vi "STEP SPEED SEQUENCE.vi"(8 "error in (no error)":errorcluster, 11 "main ref":T1) -> (0 "error out":errorcluster)   [LabVIEW 2025]
uses:
  controls/LAB-IQ UI Data.ctl
  Traction Loop/Traction Receipe Enum.ctl
  STEP SPEED SEQUENCE ENUM.ctl
  SWAY vi's/Sway Write enum.ctl
  LOAD CELL CODE/STEP LOAD SEQUENCE ENUM.ctl
  cef93557-1e48-4b46-994d-460df1ebe7ff.vi
  HEAVE vi's/Heave Write enum.ctl
panel:
  in  "Checkbox":bool
  out "ELAPSED TIMER":dbl
  out "Test Size":i32
  in  "Time Index":i32
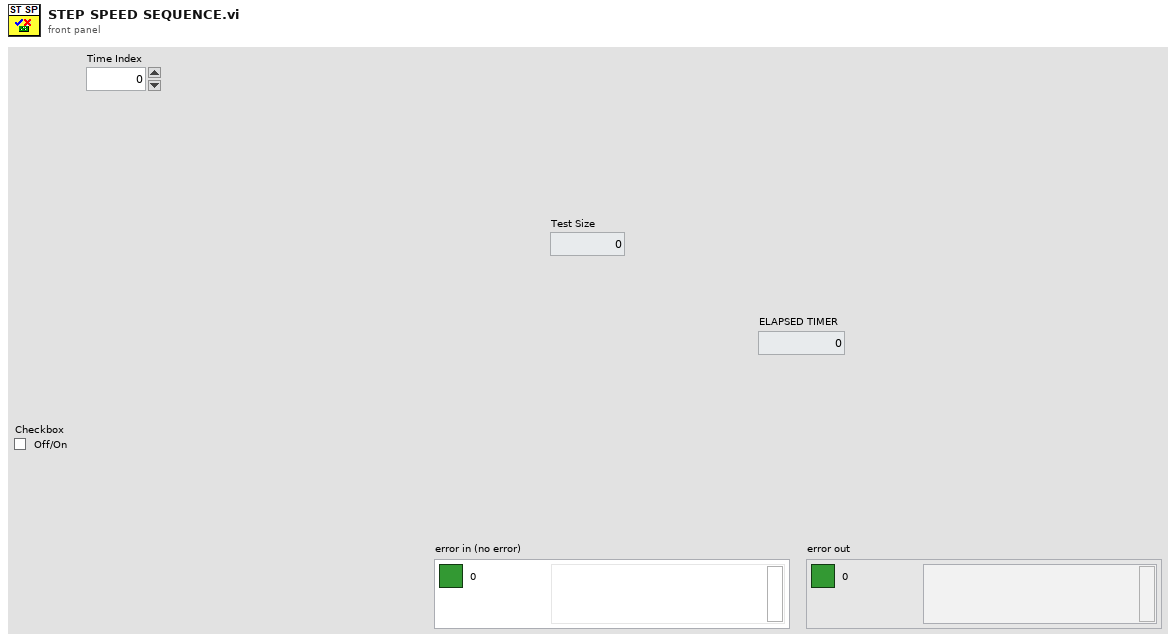
[diagram p1: front panel]
types:
  T1 = typedef "LAB-IQ UI Data.ctl" = cluster{"Main Home Screen":cluster{"GUI":refnum<vi>, "Platform Settings":refnum<vi>, "Configure":refnum<vi>, "Home":refnum<vi>, "EXIT":refnum<vi>, "service 2":refnum<vi>, "MainPage":refnum<vi>, "Analysis":refnum<vi>}, "Platform Settings":cluster{"mm/s  Surge":refnum<vi>, "Update Surge Speed":refnum<vi>, "Drive Error":refnum<vi>, "Disable Axis Jog Soft Limits":refnum<vi>, "mm/s  Sway":refnum<vi>, "Sway and Surge COM Status":refnum<vi>, "Heave COM Status":refnum<vi>, "Enable Platform":refnum<vi>, "Surge Forward Main":refnum<vi>, "Sway Right Main":refnum<vi>, "Sway Left Main":refnum<vi>, "Heave Down Main":refnum<vi>, "Heave Up main":refnum<vi>, "Update Sway Speed":refnum<vi>, "Update Heave Speed":refnum<vi>, "mm/s Heave":refnum<vi>, "mm/sec":refnum<vi>, "mm":refnum<vi>, "Surge Backward Main":refnum<vi>}, "Analysis Screen":cluster{"Analysis Home":refnum<vi>, "Surface Analysis":refnum<vi>, "Imaging":refnum<vi>, "Image Analysis":refnum<vi>, "Post Analysis":refnum<vi>}, "Config Screen":cluster{"Select Load Head":refnum<vi>, "Notes :":refnum<vi>, "FILE":refnum<vi>, "Sample ID :":refnum<vi>, "Operator ID :":refnum<vi>, "Operator Name :":refnum<vi>, "Auto":refnum<vi>}, "Motion Module":cluster{"zNL":refnum<vi>, "NL disp":refnum<vi>, "Rotary Tab":refnum<vi>, "Motion Direction:  3":refnum<vi>, "E.Velocity 2":refnum<vi>, "e.v/ssr 2":refnum<vi>, "Enter Fixed E.Velocity 2":refnum<vi>, "Enter Final SRR 2":refnum<vi>, "Enter initial SRR 2":refnum<vi>, "Enter Fixed SRR 2":refnum<vi>, "Enter the Final E.Velocity (m/s) 2":refnum<vi>, "Enter initial E.Velocity (m/s) 2":refnum<vi>, "Final Speed (RPM) 3":refnum<vi>, "Initial Speed (RPM) 2":refnum<vi>, "Enter the Final Velocity (m/s) 3":refnum<vi>, "Enter initial Velocity (m/s)  3":refnum<vi>, "Ramp Up 2":refnum<vi>, "TEST SELECTION":refnum<vi>, "SPEED SELECTION : ":refnum<vi>, "Angular Oscillation Set":refnum<vi>, "Traction":refnum<vi>, "Step Speed":refnum<vi>, "StepTable For Load-Speed":refnum<vi>, "StepTable For Speed":refnum<vi>, "Surge Forward MM":refnum<vi>, "Surge Backward MM":refnum<vi>, "M3 Image":refnum<vi>, "String 39":refnum<vi>, "Sway Left MM":refnum<vi>, "Sway Right MM":refnum<vi>, "Disable Axis Jog Soft Limits":refnum<vi>, "mm":refnum<vi>, "Heave Down MM":refnum<vi>, "Heave Up MM":refnum<vi>, "Wear Track Diameter (mm)":refnum<vi>, "Set WTD":refnum<vi>, "HomeScratch":refnum<vi>, "HomeRot":refnum<vi>, "PlaceModule":refnum<vi>, "Enter the Angle (Deg)":refnum<vi>, "Enter the Frequency (Hz)":refnum<vi>, "Motion Mode:":refnum<vi>, "LR Sway":refnum<vi>, "Rot Hor":refnum<vi>, "Scratch":refnum<vi>, "LR Cam":refnum<vi>, "MMBack":refnum<vi>, "MMNext":refnum<vi>, "Rot Ver":refnum<vi>, "Rotary Module Selection":refnum<vi>, "calculate rotary":refnum<vi>, "SPEED SELECTION : rotary":refnum<vi>, "Import 2":refnum<vi>, "Save 2":refnum<vi>, "File Path :  2":refnum<vi>, "String 45":refnum<vi>, "StepTable For Speed 3":refnum<vi>, "Enter the Speed(mm/sec)":refnum<vi>, "Enter the Speed(RPM)":refnum<vi>, "Enter Scratch Speed (mm/s):":refnum<vi>, "SwaySpeed Set":refnum<vi>, "Scartch Offset":refnum<vi>, "Motion type:":refnum<vi>, "HomeScratch 2":refnum<vi>, "Enter Scratch length (mm):":refnum<vi>, "Wear Track Diameter":refnum<vi>, "Rotary Speed Exced":refnum<vi>, "Scratch Mode":refnum<vi>, "No of Scratch":refnum<vi>}, "Environmental control":cluster{"Humidity  Status  3":refnum<vi>, "Low Temp  Status  2":refnum<vi>, "TK4 status 2":refnum<vi>, "Stage Temperature":refnum<vi>, "Sample Temperature":refnum<vi>, "Humidity (Amb)":refnum<vi>, "Clear List":refnum<vi>, "Add to list":refnum<vi>, "Wear":refnum<vi>, "Vibration":refnum<vi>, "Humidity (Chamber)":refnum<vi>, "Temperature (Chamber)":refnum<vi>, "ECR ":refnum<vi>, "Temperature (Amb)":refnum<vi>, "Microphone":refnum<vi>, "Acoustic Emission 3":refnum<vi>, "SNext":refnum<vi>, "APBack":refnum<vi>, "Enter the Temperature (°C):":refnum<vi>, "Enter the Stage \nTemperature (°C):":refnum<vi>, "Enter the Humidity (%Rh):":refnum<vi>, "Low Temp":refnum<vi>, "High Temp":refnum<vi>, "Humidity":refnum<vi>, "Sensors Picked":refnum<vi>}, "About Screen":cluster{"Password":refnum<vi>, "Home Service":refnum<vi>, "Advanced Setting":refnum<vi>, "About Tab":refnum<vi>, "ECR Port:":refnum<vi>, "Ramp Port:":refnum<vi>, "Installation/Replacement completed":refnum<vi>, "Loahead":refnum<vi>, "Heave and Surge COM Port:":refnum<vi>, "Sway COM Port:":refnum<vi>, "Temp Modbus:":refnum<vi>, "Humidity Port:":refnum<vi>, "Edit Gain Constants":refnum<vi>, "Save Gain Constants":refnum<vi>}, "Main Screen":cluster{"Main Screen Tab":refnum<vi>, "Angle and Frequency":refnum<vi>, "Stroke (mm)":refnum<vi>, "Angle (Deg)":refnum<vi>, "Main Speed Tab":refnum<vi>, "MTM MOTOR DISPLAY":refnum<vi>, "Disc Speed (m/sec)":refnum<vi>, "Ball Speed (m/sec)":refnum<vi>, "Disc Speed (RPM)":refnum<vi>, "Ball Speed (RPM)":refnum<vi>, "SPEED TAB":refnum<vi>, "Speed (m/sec)":refnum<vi>, "Set Speed (m/sec)":refnum<vi>, "Speed (RPM)":refnum<vi>, "Set Speed":refnum<vi>, "Time Tab":refnum<vi>, "Time ( HH:MM:SS ) 2":refnum<vi>, "Test Duration":refnum<vi>, "Test Duration 4":refnum<vi>, "TEST CYCLE":refnum<vi>, "TOTAL CYCLES":refnum<vi>, "Set Load (N)":refnum<vi>, "Temp Tabs":refnum<vi>, "Heater":refnum<vi>, "TK4 status":refnum<vi>, "ChamberTemp":refnum<vi>, "SetTmp":refnum<vi>, "Controller  Status":refnum<vi>, "ChamberTemp 2":refnum<vi>, "SetTmp 2":refnum<vi>, "Controller  Status 2":refnum<vi>, "ChamberTemp 3":refnum<vi>, "SetTmp 3":refnum<vi>, "Cooling":refnum<vi>, "Load Communication":refnum<vi>, "Ambient \nTemperature":refnum<vi>, "HumCOMStatus":refnum<vi>, "Ambient\n Humidity":refnum<vi>, "Freq (Hz)":refnum<vi>, "Load En":refnum<vi>, "NLt":refnum<vi>, "zNL 2":refnum<vi>, "Humidity On":refnum<vi>, "humidity disp":refnum<vi>, "Set Humidity":refnum<vi>, "NL disp 2":refnum<vi>, "Humidity On 2":refnum<vi>, "humidity disp 2":refnum<vi>, "Set Humidity 2":refnum<vi>, "NL disp 3":refnum<vi>, "AppLoadSeq scratch":refnum<vi>, "Stop Scratch":refnum<vi>, "ClrLog":refnum<vi>, "Trip Log":refnum<vi>, "STOP":refnum<vi>, "Start Test":refnum<vi>, "Test status":refnum<vi>, "AR Led":refnum<vi>, "Data":refnum<vi>, "Health":refnum<vi>, "Sway COM Status":refnum<vi>, "Heave COM Status":refnum<vi>, "Grp Tab":refnum<vi>, "Sub Graph":refnum<vi>, "SD (mm)":refnum<vi>, "Siliding distance Reset Graph":refnum<vi>, "SDGp":refnum<vi>, "Humidity Reset Graph":refnum<vi>, "HumrGp":refnum<vi>, "Acoustic Emission (mV)":refnum<vi>, "Aqucostic Reset Graph":refnum<vi>, "gACQUOS":refnum<vi>, "ECR RESET":refnum<vi>, "ECR":refnum<vi>, "Temperature Reset":refnum<vi>, "Acoustic Emission (mV) 2":refnum<vi>, "Aqucostic Reset Graph 2":refnum<vi>, "gACQUOS 2":refnum<vi>, "ECR RESET 2":refnum<vi>, "ECR 2":refnum<vi>, "Temperature Reset 2":refnum<vi>, "Temperature (deg c)":refnum<vi>, "Speed Reset Graph":refnum<vi>, "Speed Tab":refnum<vi>, "MTM DISC  SPEED":refnum<vi>, "MTM BALL SPEED":refnum<vi>, "speed mm/sec":refnum<vi>, "Hymidity":refnum<vi>, "Humidity Disable trip":refnum<vi>, "CoF Trip  2":refnum<vi>, "Depth Trip":refnum<vi>, "Weart Deapth":refnum<vi>, "Depth Reset Graph":refnum<vi>, "Weart":refnum<vi>, "Depthz":refnum<vi>, "Depth (µm)":refnum<vi>, "WearGp":refnum<vi>, "NL Trip 2":refnum<vi>, "Load pid":refnum<vi>, "Load Disable Trip":refnum<vi>, "Load Reset Graph":refnum<vi>, "NL Display 4":refnum<vi>, "Main Chart 3":refnum<vi>, "BACK":refnum<vi>, "Depth Trip 2":refnum<vi>, "COF TRIP ":refnum<vi>, "Friction Force (N)":refnum<vi>, "FF Reset Graph":refnum<vi>, "FF Disable Trip":refnum<vi>, "FF TRIP":refnum<vi>, "COF Disable Trip":refnum<vi>, "COF Reset Graph":refnum<vi>, "Start Test Temp":refnum<vi>, "zFF":refnum<vi>, "Friction Force (N) Graph":refnum<vi>, "Coefficient of Friction":refnum<vi>, "Scratch Start Test":refnum<vi>, "FF Tab":refnum<vi>, "Cyclic Friction Force (N)":refnum<vi>, "CZ FF":refnum<vi>, "Cyclic Friction Force (N) Graph":refnum<vi>, "Cyclic Coefficient of Friction":refnum<vi>, "Cyclic FF TRIP":refnum<vi>, "Cyclic FF Disable Trip":refnum<vi>, "cyclic COF Disable Trip":refnum<vi>, "cyclic COF TRIP":refnum<vi>, "cyclic COF Reset Graph":refnum<vi>, "Cyclic FF Reset Graph":refnum<vi>, "Test Trip":refnum<vi>, "Multi Scratch Pass":refnum<vi>, "Scratch Start Recording":refnum<vi>}, "Loading":cluster{"Indentation":refnum<vi>, "Reference Sample":refnum<vi>, "Load Cell Communication Slide":refnum<vi>, "com 3":refnum<vi>, "com":refnum<vi>, "DecaForce COM Status":refnum<vi>, "Update":refnum<vi>, "Clear 3":refnum<vi>, "seq":refnum<vi>, "Stribeck table":refnum<vi>, "Stribeck Table  For loading":refnum<vi>, "Loading Mode":refnum<vi>, "Enter the Final Load (N)":refnum<vi>, "Enter the CoF Trip":refnum<vi>, "Enter the Friction Force Trip":refnum<vi>, "Enter the Normal load Trip":refnum<vi>, "Enter the Load  (N)":refnum<vi>, "KiloForce":refnum<vi>, "DecaForce ":refnum<vi>, "MicroForce":refnum<vi>, "LHBack":refnum<vi>, "LHNext":refnum<vi>, "Enter the Loading Rate (N/min)":refnum<vi>, "Message":refnum<vi>, "Warning 2":refnum<vi>, "SSP 0.75":refnum<vi>, "SSP 0.5":refnum<vi>, "SSP 0.3":refnum<vi>, "Warning":refnum<vi>, "gui GIF":refnum<vi>, "Communication is established":refnum<vi>, "AppLoad 4":refnum<vi>, "Multipoint":refnum<vi>, "Load Selection":refnum<vi>}, "PID":cluster{"Ramp MulFac":refnum<vi>, "pulses LoadDiffRamp(2..10)":refnum<vi>, "PulseControlRamp(diff<=3N)":refnum<vi>, "SetLoadDeadband(%) Load(0-10N)":refnum<vi>, "PID gains out delay (microForce)":refnum<vi>, "Ramp":refnum<vi>, "Gain 2":refnum<vi>, "pulses LoadDiff(2..10)":refnum<vi>, "pulses LoadDiff(11..50)":refnum<vi>, "PulseControl(diff<=3N)":refnum<vi>, "SetLoadDeadband(%)  2":refnum<vi>, "Dummy Run":refnum<vi>, "Vertical load (N)":refnum<vi>, "AutoTune":refnum<vi>, "Offset 3 ":refnum<vi>, "apply load":refnum<vi>, "Offset  3":refnum<vi>, "apply load 2":refnum<vi>, "Enter ByPass Load":refnum<vi>, "reinit 3":refnum<vi>, "output range delay":refnum<vi>, "PID gains out delay":refnum<vi>, "Bypass Load":refnum<vi>, "pulsesSent":refnum<vi>, "pulses ":refnum<vi>, "actpid":refnum<vi>, "gFF Rot":refnum<vi>, "pulses LoadDiff(21..1000)":refnum<vi>, "Delay":refnum<vi>, "deadband":refnum<vi>}, "Config Parameters":cluster{"Tab Control 3":refnum<vi>, "Tab Control 19":refnum<vi>, "SAMPLES":refnum<vi>, "Re-initilaize":refnum<vi>, "Filter ON/OFF":refnum<vi>, "TracHomeSurgeOffsetCounts 10MM":refnum<vi>, "TracHomeSwayOffsetCounts 10MM":refnum<vi>, "Acoustic Emission:":refnum<vi>, "Apply Filter (FF)":refnum<vi>, "Filter% 2":refnum<vi>, "Apply Filter (Load)":refnum<vi>, "Filter% ":refnum<vi>, "Sway distance (mm)":refnum<vi>, "Surge distance (mm)":refnum<vi>, "DataSavingLoopDelay(ms)":refnum<vi>, "SAVE 2":refnum<vi>, "Enter Distance":refnum<vi>, "Sway Counts:":refnum<vi>, "Distance (mm): 3":refnum<vi>, "Surge Counts:":refnum<vi>, "Distance (mm): 2":refnum<vi>, "Distance (mm):":refnum<vi>, "Heave Counts:":refnum<vi>, "LRMHomeSurgeOffsetCounts":refnum<vi>, "LRMHomeSwayOffsetCounts":refnum<vi>, "TracHomeSurgeOffsetCounts 20MM":refnum<vi>, "TracHomeSwayOffsetCounts 20MM":refnum<vi>, "RotHomeSwayOffsetCounts":refnum<vi>, "RotHomeSurgeOffsetCounts":refnum<vi>, "Heave distance":refnum<vi>, "Zmm":refnum<vi>, "Heave Pulses/mm":refnum<vi>, "Surge Pulses/mm":refnum<vi>, "Sway Pulses/mm":refnum<vi>, "Heave Pitch":refnum<vi>, "Surge Pitch":refnum<vi>, "Sway Pitch":refnum<vi>, "Heave PPR":refnum<vi>, "Surge PPR":refnum<vi>, "Sway PPR":refnum<vi>, "Tab Control 5":refnum<vi>, "Tab Control 14":refnum<vi>, "Tab Control 26":refnum<vi>, "AE":refnum<vi>, "Heave Loop Delay":refnum<vi>, "Heave PID Speed":refnum<vi>, "Surge Jog Speed":refnum<vi>, "Heave Jog Speed":refnum<vi>, "Sway Loop Delay":refnum<vi>, "Sway PID Speed":refnum<vi>, "Sway Jog Speed":refnum<vi>, "DEPTH TRIP VALUE":refnum<vi>, "LOAD TRIP VALUE":refnum<vi>, "DEPTH TRIP   ENABLE":refnum<vi>, "LOAD TRIP  ENABLE":refnum<vi>, "CYCLIC FF TRIP VALUE":refnum<vi>, "FF TRIP VALUE":refnum<vi>, "CYCLIC CoF TRIP VALUE":refnum<vi>, "COF TRIP VALUE":refnum<vi>, "CYCLIC COF TRIP  ENABLE":refnum<vi>, "CYCLIC FF TRIP  ENABLE":refnum<vi>, "FF TRIP  ENABLE":refnum<vi>, "COF TRIP  ENABLE":refnum<vi>, "JOG TRIP LOAD VALUE (N)":refnum<vi>}, "Loading Com Port":cluster{"ClearAll":refnum<vi>, "Mz(Nm)":refnum<vi>, "My(Nm)":refnum<vi>, "Mx(Nm)":refnum<vi>, "Save Dwell":refnum<vi>, "Mx ":refnum<vi>, "My ":refnum<vi>, "Mz":refnum<vi>, "Fx(N)":refnum<vi>, "Fy(N)":refnum<vi>, "Fz(N)":refnum<vi>, "ZeroAll":refnum<vi>, "Acq Delay (ms)":refnum<vi>, "Burst Delay (ms)":refnum<vi>, "model":refnum<vi>, "SN":refnum<vi>, "FFx(N)":refnum<vi>, "Sensor IP":refnum<vi>, "Port":refnum<vi>, "FFy(N)":refnum<vi>, "Load(N)":refnum<vi>, "delete Handle":refnum<vi>, "Create Handle":refnum<vi>, "ft_data":refnum<vi>, "ft_range":refnum<vi>, "ft_data 2":refnum<vi>, "stop 6":refnum<vi>, "running_flag":refnum<vi>, "ft_udp_handle":refnum<vi>, "get-data-return":refnum<vi>, "get-range-return":refnum<vi>, "zero-return":refnum<vi>, "filter-return":refnum<vi>, "initial-return":refnum<vi>, "deleteHandle-result":refnum<vi>, "Load Cell Temp":refnum<vi>}, "Heave AND Surge":cluster{"SURGE POSE":refnum<vi>, "error out Read":refnum<vi>, "HEAVE POSE":refnum<vi>, "State":refnum<vi>, "Homed":refnum<vi>, "Sequence ID":refnum<vi>, "error out Write":refnum<vi>, "faultCode":refnum<vi>, "Ack ID":refnum<vi>, "SPEED":refnum<vi>, "Distance":refnum<vi>, "Mode Command":refnum<vi>, "Heave and Surge Read":refnum<vi>, "Read Heave Temp":refnum<vi>, "Spare 15":refnum<vi>, "Spare 14":refnum<vi>, "Spare 13":refnum<vi>, "Spare 12":refnum<vi>, "Spare 11":refnum<vi>, "Spare 10":refnum<vi>, "Spare 9":refnum<vi>, "Spare 8":refnum<vi>, "Spare 7":refnum<vi>, "Spare 6":refnum<vi>, "Spare 5":refnum<vi>, "Spare 4":refnum<vi>, "Spare 2":refnum<vi>, "Spare 1":refnum<vi>, "Node Id":refnum<vi>, "Spare 3":refnum<vi>, "SPARE 4":refnum<vi>, "SPARE 3":refnum<vi>, "SPARE 2":refnum<vi>, "SPARE 1":refnum<vi>, "fwMajor":refnum<vi>, "fwMinor":refnum<vi>, "Manual Write":refnum<vi>, "Heave and Surge Write":refnum<vi>, "SPARE 5":refnum<vi>, "Reserved ":refnum<vi>, "SPARE 8":refnum<vi>, "SPARE 6":refnum<vi>, "SPARE 7":refnum<vi>, "SPARE 17":refnum<vi>, "SPARE 16":refnum<vi>, "SPARE 15":refnum<vi>, "SPARE 14":refnum<vi>, "SPARE 13":refnum<vi>, "SPARE 12":refnum<vi>, "SPARE 11":refnum<vi>, "SPARE 10":refnum<vi>, "SPARE 9":refnum<vi>, "System UPTIME":refnum<vi>, "Missed Packets":refnum<vi>, "faultCode Surge Right":refnum<vi>, "faultCode Surge Left":refnum<vi>, "faultCode Heave":refnum<vi>}, "New PID LOGIC":cluster{"Fine Tune Zone":refnum<vi>, "PID SDelay":refnum<vi>, "Max_pos_limit":refnum<vi>, "Min_pos_limit":refnum<vi>, "i_limit":refnum<vi>, "pct_scale":refnum<vi>, "Deadband":refnum<vi>, "Kd":refnum<vi>, "Ki":refnum<vi>, "Kp":refnum<vi>, "Current Position":refnum<vi>, "Set Load":refnum<vi>, "Current Load":refnum<vi>, "Pulse delta":refnum<vi>, "Init Step":refnum<vi>, "Max Step Linit":refnum<vi>, "min_deadband_floor":refnum<vi>, "dynamic_spindle_noise_scalar":refnum<vi>, "min_finetune_floor":refnum<vi>, "filter_alpha":refnum<vi>}, "SWAY ":cluster{"fwMajor":refnum<vi>, "Homed":refnum<vi>, "Rotary POSE":refnum<vi>, "State":refnum<vi>, "SWAY POSE":refnum<vi>, "Ack ID":refnum<vi>, "faultCode":refnum<vi>, "Node Id":refnum<vi>, "fwMinor":refnum<vi>, "Spare 6":refnum<vi>, "Spare 5":refnum<vi>, "Spare 4":refnum<vi>, "Spare 3":refnum<vi>, "Spare 2":refnum<vi>, "Spare 1":refnum<vi>, "Spare 7":refnum<vi>, "SPARE  5":refnum<vi>, "error out Write  SWAY ":refnum<vi>, "error out Read SWAY ":refnum<vi>, "Manual Write SWAY ":refnum<vi>, "SWAY WRITE":refnum<vi>, "SPARE  4":refnum<vi>, "SPARE  3":refnum<vi>, "SPARE 2":refnum<vi>, "SPARE 1":refnum<vi>, "Spare 15":refnum<vi>, "Spare 14":refnum<vi>, "Spare 13":refnum<vi>, "Spare 12":refnum<vi>, "Spare 11":refnum<vi>, "Spare 9":refnum<vi>, "Spare 8":refnum<vi>, "SPEED":refnum<vi>, "Distance":refnum<vi>, "Mode Command":refnum<vi>, "Sequence ID":refnum<vi>, "SWAY READ":refnum<vi>, "Spare 10":refnum<vi>, "Read SWAY Temp":refnum<vi>, "faultCode Sway ":refnum<vi>, "Missed Packets":refnum<vi>, "System UPTIME sway":refnum<vi>, "SPARE 6":refnum<vi>, "SPARE 7":refnum<vi>, "SPARE 9":refnum<vi>, "SPARE 11":refnum<vi>, "SPARE 10":refnum<vi>, "SPARE 8":refnum<vi>, "SPARE 13":refnum<vi>, "SPARE 12":refnum<vi>, "SPARE 17":refnum<vi>, "SPARE 16":refnum<vi>, "SPARE 15":refnum<vi>, "SPARE 14":refnum<vi>, "Reserved":refnum<vi>, "faultCode Rotary":refnum<vi>}, "Analysis Screen":cluster{"Analysis Home":refnum<vi>, "Refresh 2":refnum<vi>, "MEAN 4":refnum<vi>, "SD 4":refnum<vi>, "VARIANCE 4":refnum<vi>, "MEAN  3":refnum<vi>, "SD  3":refnum<vi>, "VARIANCE  3":refnum<vi>, "MEAN 2":refnum<vi>, "SD  2":refnum<vi>, "VARIANCE 2":refnum<vi>, "MEAN":refnum<vi>, "SD":refnum<vi>, "VARIANCE":refnum<vi>, "File 4 Discription":refnum<vi>, "OPEN 4":refnum<vi>, "File Name 4":refnum<vi>, "OPEN 3":refnum<vi>, "File 3 Discription":refnum<vi>, "File Name 3":refnum<vi>, "Y-AXIS":refnum<vi>, "X-AXIS":refnum<vi>, "XY Graph":refnum<vi>, "File Name 2":refnum<vi>, "File Name 1":refnum<vi>, "OPEN 2":refnum<vi>, "OPEN 1":refnum<vi>, "File 1 Discription ":refnum<vi>, "File 2 Discription":refnum<vi>, "Export":refnum<vi>, "File Format":refnum<vi>}, "Traction":cluster{"faultCode Traction 2":refnum<vi>, "faultCode Traction 1":refnum<vi>, "Missed Packets":refnum<vi>, "System UPTIME Traction":refnum<vi>, "SPARE 17":refnum<vi>, "SPARE 16":refnum<vi>, "SPARE 15":refnum<vi>, "SPARE 14":refnum<vi>, "SPARE 13":refnum<vi>, "SPARE 12":refnum<vi>, "SPARE 11":refnum<vi>, "SPARE 10":refnum<vi>, "SPARE 9":refnum<vi>, "SPARE 8":refnum<vi>, "SPARE 7":refnum<vi>, "SPARE 6":refnum<vi>, "Reserved":refnum<vi>, "SPARE  5":refnum<vi>, "Manual Write TRACTION":refnum<vi>, "TRACTION WRITE":refnum<vi>, "SPARE  4":refnum<vi>, "SPARE  3":refnum<vi>, "SPARE 2":refnum<vi>, "SPARE 1":refnum<vi>, "Spare 7":refnum<vi>, "Spare 6":refnum<vi>, "Spare 5":refnum<vi>, "Spare 4":refnum<vi>, "Spare 2":refnum<vi>, "Spare 1":refnum<vi>, "Node Id":refnum<vi>, "Read TRACTION Temp":refnum<vi>, "fwMinor":refnum<vi>, "fwMajor":refnum<vi>, "faultCode":refnum<vi>, "TRACTION POSE":refnum<vi>, "TRACTION POSE 2":refnum<vi>, "Homed":refnum<vi>, "State":refnum<vi>, "Ack ID":refnum<vi>, "SPEED":refnum<vi>, "Distance":refnum<vi>, "Mode Command":refnum<vi>, "Sequence ID":refnum<vi>, "error out Read TRACTION":refnum<vi>, "error out Write  TRACTION":refnum<vi>, "TRACTION READ":refnum<vi>, "Spare 3":refnum<vi>}, "Traction reciepe":cluster{"SRR Sweep Range (%) Stribeck":refnum<vi>, "Traction Receipe":refnum<vi>, "Total Execution Time":refnum<vi>, "Total Steps":refnum<vi>, "Duration / Step (s)  Stribeck":refnum<vi>, "STRIBECK Fixed SRR List (%)":refnum<vi>, "Duration / Step (s) Traction":refnum<vi>, "SRR Sweep Range (%) traction":refnum<vi>, "Rolling Speed (mm/s)":refnum<vi>, "Temperature Stages (°C)":refnum<vi>, "Ball Load (N)":refnum<vi>, "Lubricant Name":refnum<vi>, "Profile File Name":refnum<vi>, "SET entrainment Velocity":refnum<vi>, "Test Array Size":refnum<vi>, "SRR INDEX [ STRIBECK]":refnum<vi>, "Stribeck Size":refnum<vi>, "SET SRR":refnum<vi>, "ELAPSED TIMER ":refnum<vi>, "BALL SET RPM":refnum<vi>, "DISC SET RPM":refnum<vi>, "SET LOAD":refnum<vi>, "TEMPERATURE READ":refnum<vi>, "SET TEMPERATURE":refnum<vi>, "Traction Size":refnum<vi>, "DISC SPEED (rpm)":refnum<vi>, "BALL SPEED (rpm)":refnum<vi>, "BALL WEAR TRACK":refnum<vi>, "DISC WEARTRACK":refnum<vi>, "SRR INDEX [ TRACTION]":refnum<vi>, "Start Index Type":refnum<vi>, "Enum - Menu":refnum<vi>, "Ball (mm/sec)":refnum<vi>, "Disc (mm/sec)":refnum<vi>}, "Traction Control":cluster{"HomeTraction":refnum<vi>, "Demo Mode Display":refnum<vi>, "Traction Message":refnum<vi>, "Traction Step Update Details":refnum<vi>, "Main Tab sequence for selection":refnum<vi>, "Ramp Tab":refnum<vi>, "e.v/ssr":refnum<vi>, "Enter Fixed E.Velocity":refnum<vi>, "Enter Final SRR":refnum<vi>, "Enter initial SRR":refnum<vi>, "Enter Fixed SRR":refnum<vi>, "Enter the Final E.Velocity (m/s)":refnum<vi>, "Enter initial E.Velocity (m/s)":refnum<vi>, "Ball WTD":refnum<vi>, "E.Velocity":refnum<vi>, "Enter the Final Velocity (m/s)":refnum<vi>, "Enter initial Velocity (m/s)":refnum<vi>, "Ramp Up   Disc":refnum<vi>, "Initial DiscSpeed (RPM)":refnum<vi>, "Final Speed (RPM) Ball":refnum<vi>, "Final Speed (RPM)":refnum<vi>, "Initial Speed (RPM) Ball":refnum<vi>, "Enter the Final Velocity (m/s) Ball":refnum<vi>, "Enter initial Velocity (m/s) Ball":refnum<vi>, "Ramp Up":refnum<vi>, "ExceedBallSpeed step":refnum<vi>, "ExceedDiscSpeed":refnum<vi>, "BallSpeed Exceed Indication":refnum<vi>, "Apply":refnum<vi>, "SPEED SELECTION : MTM":refnum<vi>, "SPEED SELECTION : MTM 2":refnum<vi>, "TEST SELECTION (MTM)":refnum<vi>, "MTM Test Selection":refnum<vi>, "File Path Tab":refnum<vi>, "File Path String":refnum<vi>, "Save":refnum<vi>, "Save  2":refnum<vi>, "Import ":refnum<vi>, "File Path :":refnum<vi>, "Step Sequence Indication Tab":refnum<vi>, "Step Sequence Indication":refnum<vi>, "Calculate Step":refnum<vi>, "StepTable":refnum<vi>, "ExceedDiscSpeed  Cinstant Speed":refnum<vi>, "ExceedBallSpeed Constant":refnum<vi>, "TEST SELECTION (MTM) 2":refnum<vi>, "SPEED SELECTION : MTM 3":refnum<vi>, "MTM Test Selection 2":refnum<vi>, "Enter the Speed (m/sec): ":refnum<vi>, "Enter the Speed (m/sec):  2":refnum<vi>, "Enter the Speed (RPM):":refnum<vi>, "Lower Spped ":refnum<vi>, "Upper":refnum<vi>, "Enter the Speed (RPM):Ball":refnum<vi>, "Disc Motion Direction: ":refnum<vi>, "Ball Motion Direction :":refnum<vi>, "Motion Mode: ":refnum<vi>, "Wear Track Diameter (mm) ":refnum<vi>, "Disc Speed Indicator":refnum<vi>, "ExceedBallSpeed":refnum<vi>}, "Acquostic":cluster{"Last Config Rejected ":refnum<vi>, "rx command count":refnum<vi>, "Current Filter Id":refnum<vi>, "Isolated Gain":refnum<vi>, "DAQ Status":refnum<vi>, "error out":refnum<vi>, "error in (no error)":refnum<vi>, "Uplink Packet":refnum<vi>, "data out":refnum<vi>, "Downlink Packet":refnum<vi>, "Signal Energy":refnum<vi>, "Amplitude db_AE":refnum<vi>, "Peak Amplitude":refnum<vi>, "AE Ring-Down Counts":refnum<vi>, "Gains":refnum<vi>, "Manual Write Acquostic":refnum<vi>}}
  T2 = enum32{"Setup", "Load Head", "Motion Module", "Environment", "Begin"}
  T3 = typedef "STEP SPEED SEQUENCE ENUM.ctl" = enum16{"INIT", "TEST START", "TEST INCREMENT", "TEST STOP"}
  T4 = typedef "Sway Write enum.ctl" = enum16{"INIT", "WRITE", "CLOSE", "REINIT"}
  T5 = typedef "Heave Write enum.ctl" = enum16{"INIT", "WRITE", "CLOSE", "REINIT"}
  T6 = typedef "STEP LOAD SEQUENCE ENUM.ctl" = enum16{"INIT", "TEST START", "TEST INCREMENT", "TEST STOP"}
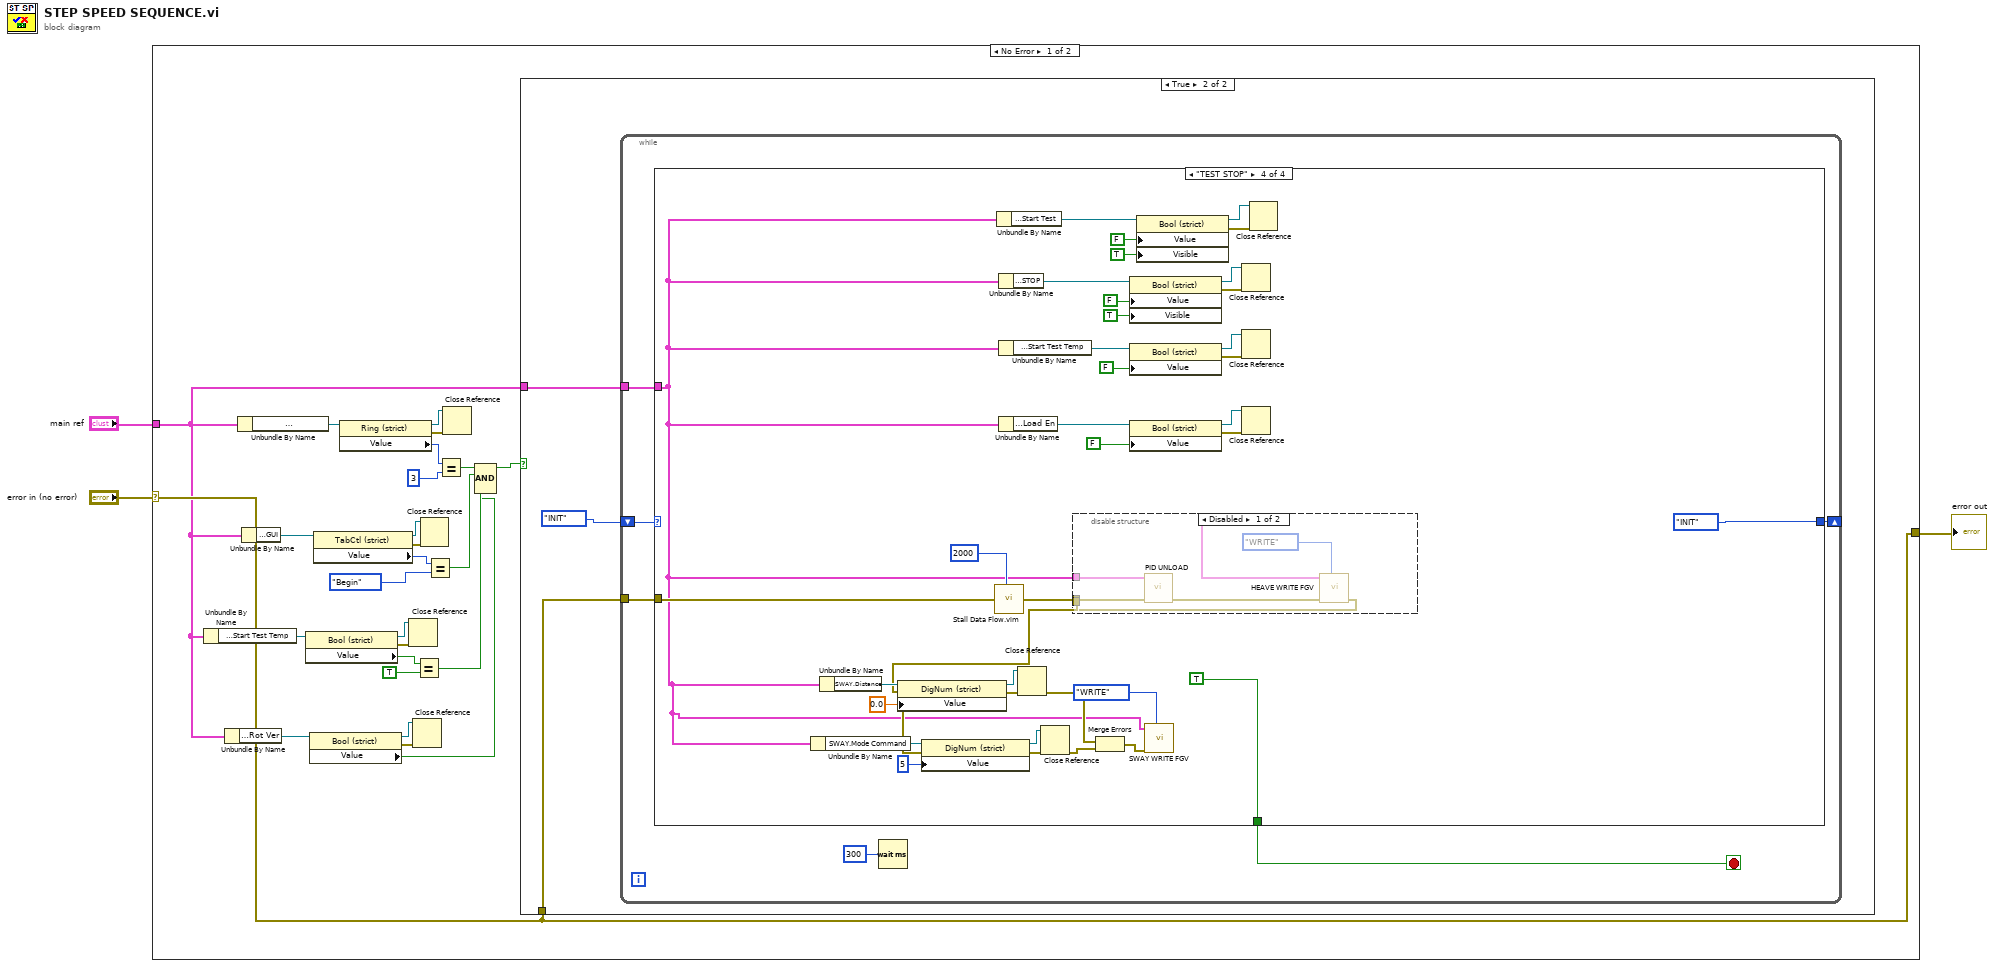
[diagram p0: block diagram]
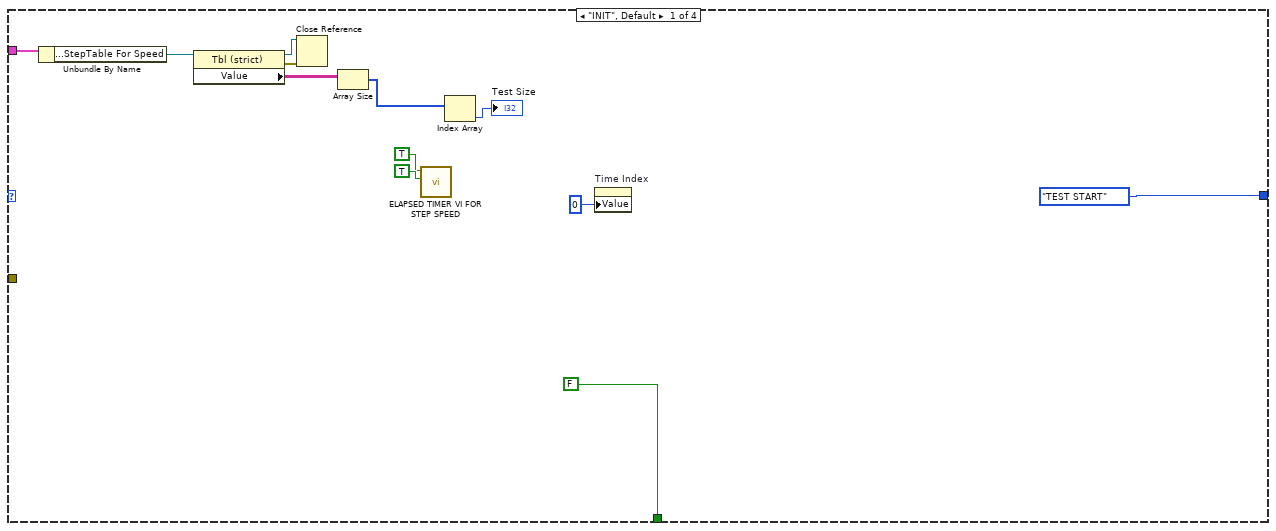
[diagram p3: hidden frame]
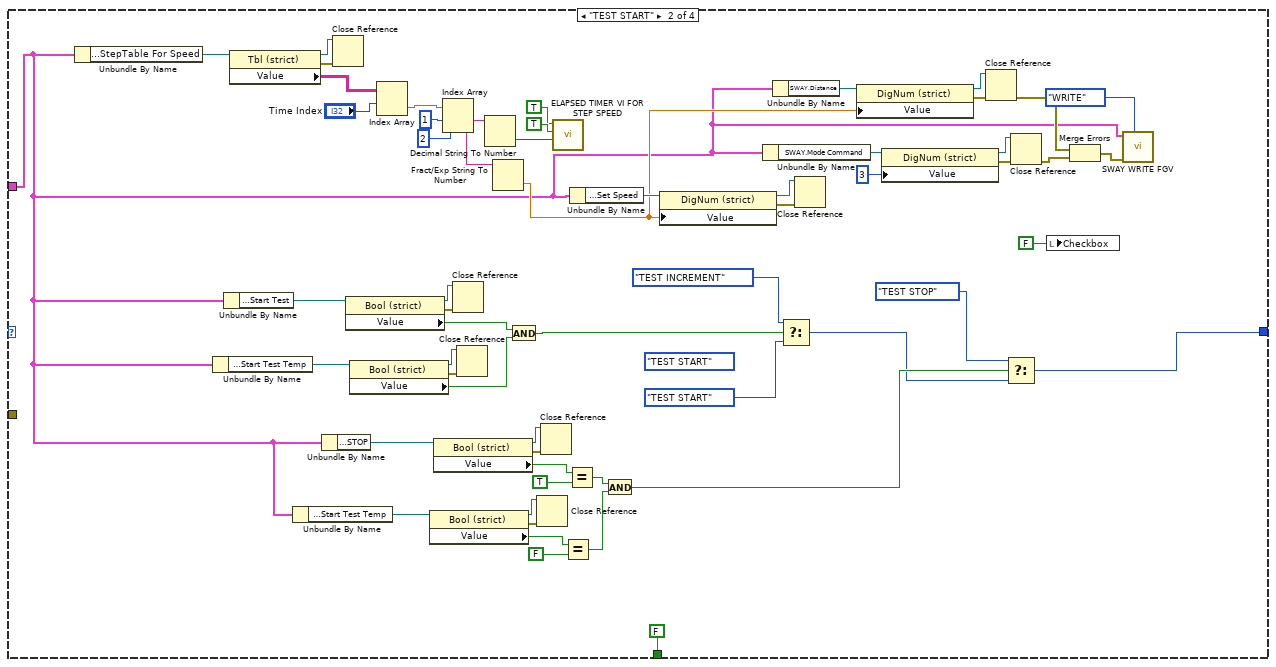
[diagram p4: hidden frame]
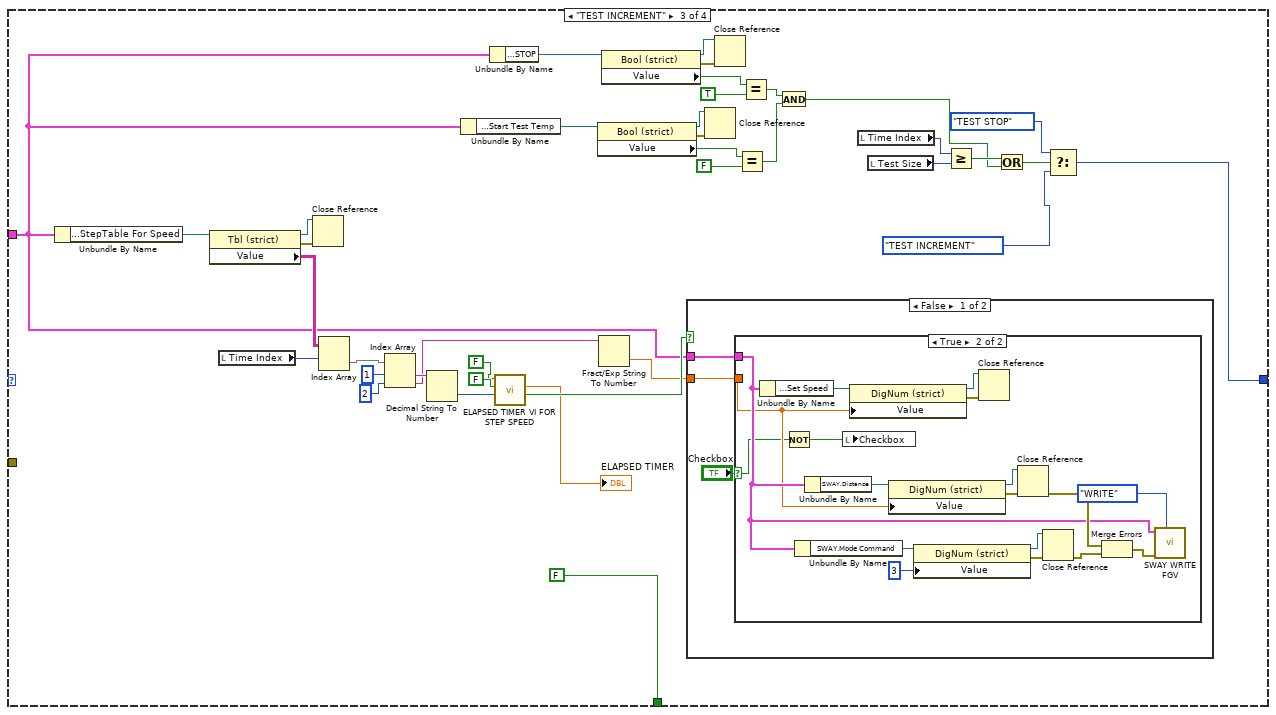
[diagram p5: hidden frame]
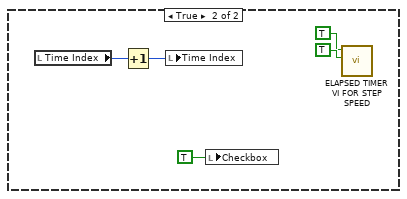
[diagram p7: hidden frame]
diagram:
  n1 = case shown="No Error" "error in (no error)" {
    selector: "error in (no error)" -> [w9 _]
    tunnel: "main ref" -> [w6 _]
    tunnel: [w9 _] -> w1
    frame No Error {
      n2 = Unbundle By Name(w6) -> ("Main Screen.Start Test Temp"=w14:refnum<vi>)
      n3 = Unbundle By Name(w6) -> ("Motion Module.Rot Ver"=w8:refnum<vi>)
      n4 = Unbundle By Name(w6) -> ("Motion Module.Motion Mode:"=w28:refnum<vi>)
      n5 = Unbundle By Name(w6) -> ("Main Home Screen.GUI"=w20:refnum<vi>)
      n6 = property class="Bool (strict)"(reference=w14) -> (reference out=w12:refnum<vi>, error out=w13:errorcluster, "Value"=w15:bool)  [unwired: 1 in]
      n7 = property class="Bool (strict)"(reference=w8) -> (reference out=w4:refnum<vi>, error out=w7:errorcluster, "Value"=w5:bool)  [unwired: 1 in]
      n8 = property class="TabCtl (strict)"(reference=w20) -> (reference out=w22:refnum<vi>, error out=w21:errorcluster, "Value"=w18:T2)  [unwired: 1 in]
      n9 = property class="Ring (strict)"(reference=w28) -> (reference out=w26:refnum<vi>, error out=w27:errorcluster, "Value"=w25:u16)  [unwired: 1 in]
      n10 = Close Reference(reference=w12, error in (no error)=w13) -> ()  [unwired: 1 out]
      n11 = Close Reference(reference=w4, error in (no error)=w7) -> ()  [unwired: 1 out]
      n12 = Equal?(x=w15, y=TRUE) -> (x = y?=w11:bool)
      n13 = Close Reference(reference=w22, error in (no error)=w21) -> ()  [unwired: 1 out]
      n14 = Equal?(x=w18, y=T2."Begin" ("Value")) -> (x = y?=w16:bool)
      n15 = Equal?(x=w25, y=u16 3 ("Value")) -> (x = y?=w23:bool)
      n16 = Close Reference(reference=w26, error in (no error)=w27) -> ()  [unwired: 1 out]
      n17 = Compound Arithmetic op=AND(w23, w16, w11, w5) -> (w19:bool)
      n18 = case shown="True" w19 {
        tunnel: w6 -> [_ w30]
        tunnel: w9 -> [_ w29]
        frame False {
        }
        frame True {
          n19 = while {
            shift-right: [w36] -> _
            shift-left: STEP_SPEED_SEQUENCE_ENUM."INIT" -> [w37]
            tunnel: w30 -> [w34]
            tunnel: w29 -> [w33]
            stop <- w35 stop-if-true
            n20 = case shown="\"TEST STOP\"" w37 {
              tunnel: [STEP_SPEED_SEQUENCE_ENUM."TEST START" w72 w130 STEP_SPEED_SEQUENCE_ENUM."INIT"] -> w36
              tunnel: [FALSE FALSE FALSE TRUE] -> w35
              tunnel: w34 -> [w40 w51 w110 w173]
              tunnel: w33 -> [_ _ _ w193]
              frame "INIT", Default {
                n21 = Unbundle By Name(w40) -> ("Motion Module.StepTable For Speed"=w43:refnum<vi>)
                n22 = property class="Tbl (strict)"(reference=w43) -> (reference out=w41:refnum<vi>, error out=w42:errorcluster, "Value"=w39:string[][])  [unwired: 1 in]
                n23 = Close Reference(reference=w41, error in (no error)=w42) -> ()  [unwired: 1 out]
                n24 = Array Size(array=w39) -> (size(s)=w46:i32[])
                n25 = call "ELAPSED TIMER VI FOR STEP SPEED.vi"("RESET"=TRUE, "PAUSE"=TRUE) -> ()  [unwired: 7 in, 3 out]
                n26 = Index Array(array=w46) -> (element=→"Test Size":i32)  [unwired: 1 in]
                n27 = property on="Time Index" class="DigNum (strict)"("Value"=0 ("Time Index")) -> ()  [unwired: 2 in, 2 out]
              }
              frame "TEST START" {
                (unwired) STEP_LOAD_SEQUENCE_ENUM."TEST START"
                n28 = Unbundle By Name(w51) -> ("Motion Module.StepTable For Speed"=w100:refnum<vi>)
                n29 = Unbundle By Name(w51) -> ("Main Screen.Start Test Temp"=w93:refnum<vi>)
                n30 = Unbundle By Name(w51) -> ("Main Screen.Start Test"=w94:refnum<vi>)
                n31 = property class="Tbl (strict)"(reference=w100) -> (reference out=w98:refnum<vi>, error out=w99:errorcluster, "Value"=w97:string[][])  [unwired: 1 in]
                n32 = Unbundle By Name(w51) -> ("Main Screen.Start Test Temp"=w80:refnum<vi>)
                n33 = Unbundle By Name(w51) -> ("Main Screen.STOP"=w85:refnum<vi>)
                n34 = Close Reference(reference=w98, error in (no error)=w99) -> ()  [unwired: 1 out]
                n35 = property class="Bool (strict)"(reference=w94) -> (reference out=w96:refnum<vi>, error out=w95:errorcluster, "Value"=w90:bool)  [unwired: 1 in]
                n36 = property class="Bool (strict)"(reference=w93) -> (reference out=w91:refnum<vi>, error out=w92:errorcluster, "Value"=w89:bool)  [unwired: 1 in]
                n37 = Index Array(array=w97, index (row)="Time Index") -> (element=w106:string[])  [unwired: 1 in]
                n38 = property class="Bool (strict)"(reference=w80) -> (reference out=w78:refnum<vi>, error out=w79:errorcluster, "Value"=w81:bool)  [unwired: 1 in]
                n39 = property class="Bool (strict)"(reference=w85) -> (reference out=w87:refnum<vi>, error out=w86:errorcluster, "Value"=w84:bool)  [unwired: 1 in]
                n40 = Index Array(array=w106, index #1=1 ("index"), index #2=2 ("index")) -> (element #1=w104:string, element #2=w67:string)
                n41 = Close Reference(reference=w96, error in (no error)=w95) -> ()  [unwired: 1 out]
                n42 = Close Reference(reference=w91, error in (no error)=w92) -> ()  [unwired: 1 out]
                n43 = Decimal String To Number(string=w104) -> (number=w101:i32)  [unwired: 2 in, 1 out]
                n44 = Fract/Exp String To Number(string=w67) -> (number=w54:dbl)  [unwired: 3 in, 1 out]
                n45 = And(x=w90, y=w89) -> (x .and. y?=w88:bool)
                n46 = Close Reference(reference=w78, error in (no error)=w79) -> ()  [unwired: 1 out]
                n47 = Close Reference(reference=w87, error in (no error)=w86) -> ()  [unwired: 1 out]
                n48 = call "ELAPSED TIMER VI FOR STEP SPEED.vi"("TARGET"=w101, "RESET"=TRUE, "PAUSE"=TRUE) -> ()  [unwired: 6 in, 3 out]
                n49 = Equal?(x=w81, y=FALSE) -> (x = y?=w76:bool)
                n50 = Equal?(x=w84, y=TRUE) -> (x = y?=w77:bool)
                n51 = Unbundle By Name(w51) -> ("Main Screen.Set Speed"=w66:refnum<vi>)
                n52 = And(x=w77, y=w76) -> (x .and. y?=w74:bool)
                n53 = property class="DigNum (strict)"(reference=w66, "Value"=w54) -> (reference out=w64:refnum<vi>, error out=w65:errorcluster)  [unwired: 1 in]
                n54 = Unbundle By Name(w51) -> ("SWAY.Mode Command"=w58:refnum<vi>)
                n55 = Unbundle By Name(w51) -> ("SWAY.Distance"=w63:refnum<vi>)
                n56 = Select(t=STEP_SPEED_SEQUENCE_ENUM."TEST INCREMENT", s=w88, f=STEP_SPEED_SEQUENCE_ENUM."TEST START") -> (s? t:f=w73:T3)
                n57 = Close Reference(reference=w64, error in (no error)=w65) -> ()  [unwired: 1 out]
                n58 = property class="DigNum (strict)"(reference=w63, "Value"=w54) -> (reference out=w61:refnum<vi>, error out=w62:errorcluster)  [unwired: 1 in]
                n59 = property class="DigNum (strict)"(reference=w58, "Value"=u8 3) -> (reference out=w60:refnum<vi>, error out=w59:errorcluster)  [unwired: 1 in]
                n60 = Close Reference(reference=w61, error in (no error)=w62) -> (error out=w55:errorcluster)
                n61 = Select(t=STEP_SPEED_SEQUENCE_ENUM."TEST STOP", s=w74, f=w73) -> (s? t:f=w72:T3)
                n62 = Close Reference(reference=w60, error in (no error)=w59) -> (error out=w56:errorcluster)
                n63 = local write "Checkbox"(FALSE ("Checkbox")) -> ()
                n64 = Merge Errors(w55, w56) -> (w53:errorcluster)
                n65 = call "SWAY WRITE FGV.vi"("Enum - Menu"=Sway_Write_enum."WRITE", "error in (no error)"=w53, "main ref"=w51) -> ()  [unwired: 8 in, 1 out]
              }
              frame "TEST INCREMENT" {
                n66 = Unbundle By Name(w110) -> ("Motion Module.StepTable For Speed"=w127:refnum<vi>)
                n67 = property class="Tbl (strict)"(reference=w127) -> (reference out=w125:refnum<vi>, error out=w126:errorcluster, "Value"=w124:string[][])  [unwired: 1 in]
                n68 = local read "Time Index"() -> (w145:i32)
                n69 = Close Reference(reference=w125, error in (no error)=w126) -> ()  [unwired: 1 out]
                n70 = Index Array(array=w124, index (row)=w145) -> (element=w140:string[])  [unwired: 1 in]
                n71 = Index Array(array=w140, index #1=1 ("index"), index #2=2 ("index")) -> (element #1=w139:string, element #2=w136:string)
                n72 = Decimal String To Number(string=w139) -> (number=w144:i32)  [unwired: 2 in, 1 out]
                n73 = Unbundle By Name(w110) -> ("Main Screen.Start Test Temp"=w116:refnum<vi>)
                n74 = Unbundle By Name(w110) -> ("Main Screen.STOP"=w121:refnum<vi>)
                n75 = call "ELAPSED TIMER VI FOR STEP SPEED.vi"("TARGET"=w144, "RESET"=FALSE, "PAUSE"=FALSE) -> ("ELAPSED INDICATION"=w138:bool, "ELAPSED TIMER"=→"ELAPSED TIMER":dbl)  [unwired: 6 in, 1 out]
                n76 = property class="Bool (strict)"(reference=w116) -> (reference out=w114:refnum<vi>, error out=w115:errorcluster, "Value"=w117:bool)  [unwired: 1 in]
                n77 = Fract/Exp String To Number(string=w136) -> (number=w129:dbl)  [unwired: 3 in, 1 out]
                n78 = property class="Bool (strict)"(reference=w121) -> (reference out=w123:refnum<vi>, error out=w122:errorcluster, "Value"=w120:bool)  [unwired: 1 in]
                n79 = case shown="False" w138 {
                  tunnel: w129 -> [w147 _]
                  tunnel: w110 -> [w148 _]
                  frame False {
                    n80 = case shown="True" "Checkbox" {
                      selector: "Checkbox" -> [_ w150]
                      tunnel: w148 -> [_ w152]
                      tunnel: w147 -> [_ w151]
                      frame False {
                      }
                      frame True {
                        n81 = Unbundle By Name(w152) -> ("Main Screen.Set Speed"=w166:refnum<vi>)
                        n82 = Not(x=w150) -> (.not. x?=w149:bool)
                        n83 = Unbundle By Name(w152) -> ("SWAY.Mode Command"=w158:refnum<vi>)
                        n84 = Unbundle By Name(w152) -> ("SWAY.Distance"=w163:refnum<vi>)
                        n85 = local write "Checkbox"(w149) -> ()
                        n86 = property class="DigNum (strict)"(reference=w166, "Value"=w151) -> (reference out=w164:refnum<vi>, error out=w165:errorcluster)  [unwired: 1 in]
                        n87 = property class="DigNum (strict)"(reference=w163, "Value"=w151) -> (reference out=w161:refnum<vi>, error out=w162:errorcluster)  [unwired: 1 in]
                        n88 = property class="DigNum (strict)"(reference=w158, "Value"=u8 3) -> (reference out=w160:refnum<vi>, error out=w159:errorcluster)  [unwired: 1 in]
                        n89 = Close Reference(reference=w164, error in (no error)=w165) -> ()  [unwired: 1 out]
                        n90 = Close Reference(reference=w161, error in (no error)=w162) -> (error out=w156:errorcluster)
                        n91 = Close Reference(reference=w160, error in (no error)=w159) -> (error out=w157:errorcluster)
                        n92 = Merge Errors(w156, w157) -> (w155:errorcluster)
                        n93 = call "SWAY WRITE FGV.vi"("Enum - Menu"=Sway_Write_enum."WRITE", "error in (no error)"=w155, "main ref"=w152) -> ()  [unwired: 8 in, 1 out]
                      }
                    }
                  }
                  frame True {
                    n94 = local read "Time Index"() -> (w171:i32)
                    n95 = Increment(x=w171) -> (x+1=w170:i32)
                    n96 = local write "Time Index"(w170) -> ()
                    n97 = local write "Checkbox"(TRUE ("Checkbox")) -> ()
                    n98 = call "ELAPSED TIMER VI FOR STEP SPEED.vi"("RESET"=TRUE, "PAUSE"=TRUE) -> ()  [unwired: 7 in, 3 out]
                  }
                }
                n99 = Close Reference(reference=w114, error in (no error)=w115) -> ()  [unwired: 1 out]
                n100 = Close Reference(reference=w123, error in (no error)=w122) -> ()  [unwired: 1 out]
                n101 = Equal?(x=w117, y=FALSE) -> (x = y?=w112:bool)
                n102 = Equal?(x=w120, y=TRUE) -> (x = y?=w113:bool)
                n103 = And(x=w113, y=w112) -> (x .and. y?=w111:bool)
                n104 = local read "Time Index"() -> (w134:i32)
                n105 = local read "Test Size"() -> (w133:i32)
                n106 = Greater Or Equal?(x=w134, y=w133) -> (x >= y?=w132:bool)
                n107 = Or(x=w132, y=w111) -> (x .or. y?=w131:bool)
                n108 = Select(t=STEP_SPEED_SEQUENCE_ENUM."TEST STOP", s=w131, f=STEP_SPEED_SEQUENCE_ENUM."TEST INCREMENT") -> (s? t:f=w130:T3)
              }
              frame "TEST STOP" {
                n109 = Unbundle By Name(w173) -> ("SWAY.Mode Command"=w180:refnum<vi>)
                n110 = Unbundle By Name(w173) -> ("SWAY.Distance"=w185:refnum<vi>)
                n111 = call "Stall Data Flow.vim"("value in"=w193, "milliseconds to wait"=u32 2000) -> ("value out"=w195:errorcluster)  [unwired: 1 out]
                n112 = Unbundle By Name(w173) -> ("Main Screen.Start Test"=w191:refnum<vi>)
                n113 = Unbundle By Name(w173) -> ("Main Screen.STOP"=w205:refnum<vi>)
                n114 = Unbundle By Name(w173) -> ("Main Screen.Start Test Temp"=w204:refnum<vi>)
                n115 = Unbundle By Name(w173) -> ("Main Screen.Load En"=w196:refnum<vi>)
                n116 = disable-structure shown="Disabled" {
                  disable-tunnel: w195 -> [w211 w214]
                  disable-tunnel: [w210 w214] -> w174
                  disable-tunnel: w173 -> [w209 _]
                  frame Disabled {
                    n117 = call "PID UNLOAD.vi"("error in (no error)"=w211, "main ref"=w209) -> ("error out"=w212:errorcluster)  [unwired: 9 in]
                    n118 = call "HEAVE WRITE FGV.vi"("Enum - Menu"=Heave_Write_enum."WRITE", "error in (no error)"=w212, "main ref"=w209) -> ("error out"=w210:errorcluster)  [unwired: 8 in]
                  }
                  frame Enabled {
                  }
                }
                n119 = property class="DigNum (strict)"(reference=w185, error in=w174, "Value"=sgl 0.0) -> (reference out=w183:refnum<vi>, error out=w184:errorcluster)
                n120 = property class="DigNum (strict)"(reference=w180, error in=w174, "Value"=u8 5) -> (reference out=w182:refnum<vi>, error out=w181:errorcluster)
                n121 = Close Reference(reference=w183, error in (no error)=w184) -> (error out=w177:errorcluster)
                n122 = Close Reference(reference=w182, error in (no error)=w181) -> (error out=w178:errorcluster)
                n123 = Merge Errors(w177, w178) -> (w176:errorcluster)
                n124 = property class="Bool (strict)"(reference=w205, "Value"=FALSE, "Visible"=TRUE) -> (reference out=w207:refnum<vi>, error out=w206:errorcluster)  [unwired: 1 in]
                n125 = property class="Bool (strict)"(reference=w204, "Value"=FALSE) -> (reference out=w202:refnum<vi>, error out=w203:errorcluster)  [unwired: 1 in]
                n126 = property class="Bool (strict)"(reference=w196, "Value"=FALSE) -> (reference out=w198:refnum<vi>, error out=w197:errorcluster)  [unwired: 1 in]
                n127 = property class="Bool (strict)"(reference=w191, "Value"=FALSE, "Visible"=TRUE) -> (reference out=w189:refnum<vi>, error out=w190:errorcluster)  [unwired: 1 in]
                n128 = call "SWAY WRITE FGV.vi"("Enum - Menu"=Sway_Write_enum."WRITE", "error in (no error)"=w176, "main ref"=w173) -> ()  [unwired: 8 in, 1 out]
                n129 = Close Reference(reference=w207, error in (no error)=w206) -> ()  [unwired: 1 out]
                n130 = Close Reference(reference=w202, error in (no error)=w203) -> ()  [unwired: 1 out]
                n131 = Close Reference(reference=w198, error in (no error)=w197) -> ()  [unwired: 1 out]
                n132 = Close Reference(reference=w189, error in (no error)=w190) -> ()  [unwired: 1 out]
              }
            }
            n133 = Wait (ms)(milliseconds to wait=u32 300) -> ()  [unwired: 1 out]
          }
        }
      }
    }
    frame Error {
    }
  }
  "error out" <- w1
